vi "flow-rate-global.vi"() -> ()   [LabVIEW 2014]
panel:
  in  "Flow Rate":dbl=100.0
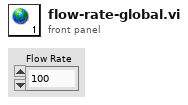
[diagram p1: front panel]
diagram:
